vi "Get Interface Status.vi"(8 "error in (no error)":errorcluster, 11 "Application in":refnum<class "Application.lvclass">) -> (0 "error out":errorcluster, 2 "RED panel Cluster":T1={"Exposing"=TRUE, "% Acquired"=0.0, "Initialization"=FALSE, "CurrentlyTemp"=0, "Exposições realizadas"=0, "Image Graph"=[], "Temperature Status"="", "Last Image"=""} {"Exposições realizadas" scale=0.0..1.0}, 3 "Application out":refnum<class "Application.lvclass">)   [LabVIEW 2018, in "Application.lvclass"]
doc: "Este VI faz a leitura do status da interface: porcentagem de exposição da imagem atual, indicador de exposição, temperatura do CCD, indicador de inicialização do CCD, número de exposições realizadas, status da temperatura (para controle da cor do background do indicador de temperatura), última imagem obtida e gráfico da última imagem."
uses:
  Application.lvclass
  Application.lvclass/Application.ctl
  CCDCamera/CCDCamera.lvclass/CCDCamera.ctl
  Cooler/Cooler.lvclass/Cooler.ctl
  CCDCamera/CCDCamera.lvclass
  Display Image/Display Image.lvclass
  Cooler/Cooler.lvclass
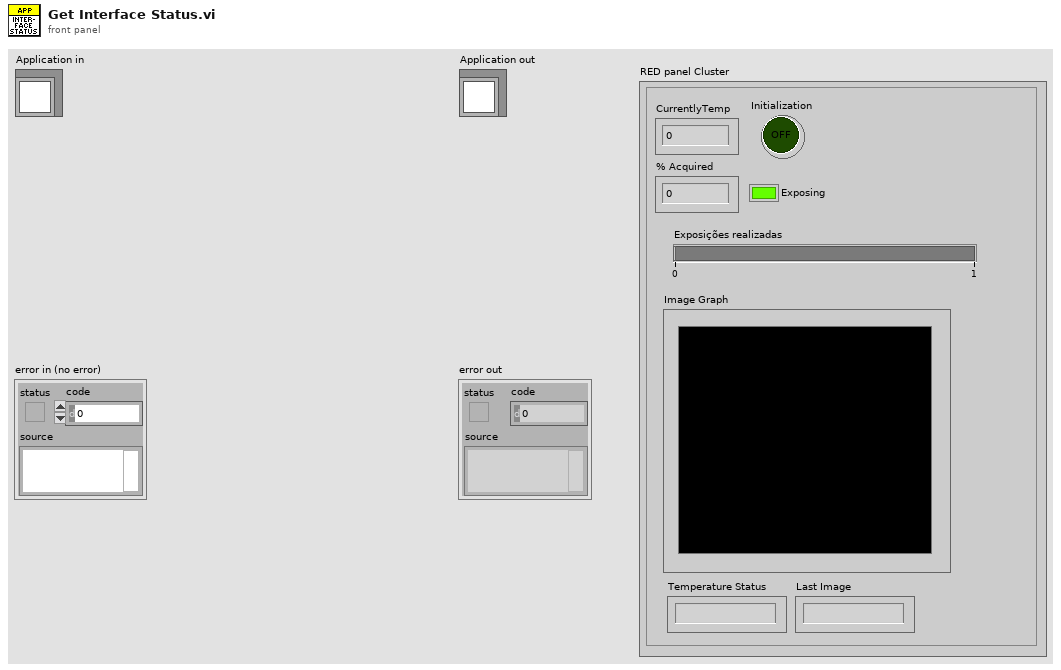
[diagram p1: front panel]
types:
  T1 = cluster{"Exposing":bool, "% Acquired":dbl, "Initialization":bool, "CurrentlyTemp":i16, "Exposições realizadas":u8, "Image Graph":i32[][], "Temperature Status":string, "Last Image":string}
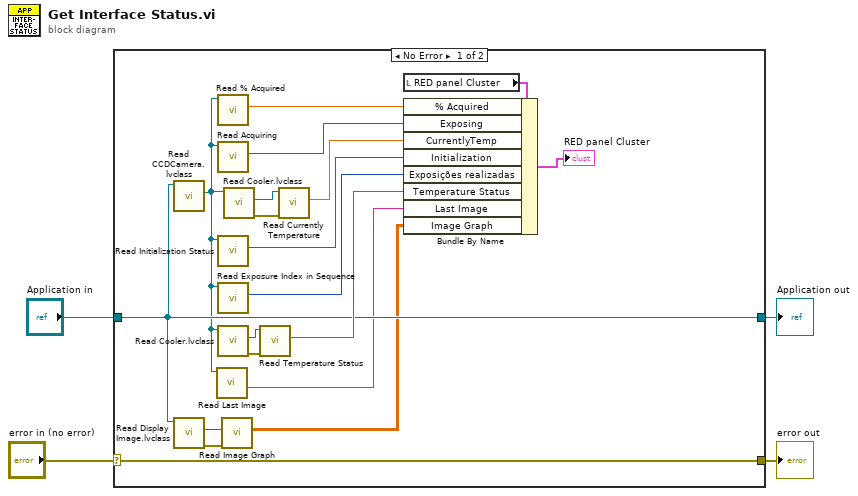
[diagram p0: block diagram]
diagram:
  n1 = case shown="No Error" "error in (no error)" {
    selector: "error in (no error)" -> [w23 w25]
    tunnel: [w23 w25] -> w3
    tunnel: [w10 w24] -> w1
    tunnel: "Application in" -> [w10 w24]
    frame No Error {
      n2 = call "Read CCDCamera.lvclass.vi"("Application in"=w10) -> ("CCDCamera.lvclass"=w6:refnum<class "CCDCamera.lvclass">)  [unwired: 8 in, 2 out]
      n3 = call "Read Display Image.lvclass.vi"("Application in"=w10) -> ("error out"=w9:errorcluster, "Display Image.lvclass"=w8:refnum<class "Display Image.lvclass">)  [unwired: 8 in, 1 out]
      n4 = call "Read Last Image.vi"("CCDCamera in"=w6) -> ("Last Image"=w5:string)  [unwired: 7 in, 3 out]
      n5 = call "Read % Acquired.vi"("CCDCamera in"=w6) -> ("% Acquired"=w21:dbl)  [unwired: 8 in, 2 out]
      n6 = call "Read Acquiring.vi"("CCDCamera in"=w6) -> ("Acquiring"=w20:bool)  [unwired: 8 in, 2 out]
      n7 = call "Read Initialization Status.vi"("CCDCamera in"=w6) -> ("Initialization Status"=w19:bool)  [unwired: 8 in, 2 out]
      n8 = call "Read Exposure Index in Sequence.vi"("CCDCamera in"=w6) -> ("Exposure Index in Sequence"=w17:u16)  [unwired: 8 in, 2 out]
      n9 = call "Read Cooler.lvclass.vi"("CCDCamera in"=w6) -> ("error out"=w16:errorcluster, "Cooler.lvclass"=w15:refnum<class "Cooler.lvclass">)  [unwired: 8 in, 1 out]
      n10 = call "Read Image Graph.vi"("error in (no error)"=w9, "Display Image in"=w8) -> ("Image Graph"=w7:dbl[][])  [unwired: 7 in, 2 out]
      n11 = call "Read Cooler.lvclass.vi"("CCDCamera in"=w6) -> ("error out"=w13:errorcluster, "Cooler.lvclass"=w12:refnum<class "Cooler.lvclass">)  [unwired: 8 in, 1 out]
      n12 = call "Read Temperature Status.vi"("error in (no error)"=w16, "Cooler in"=w15) -> ("Temperature Status"=w14:string)  [unwired: 7 in, 2 out]
      n13 = call "Read Currently Temperature.vi"("error in (no error)"=w13, "Cooler in"=w12) -> ("Currently Temperature"=w11:dbl)  [unwired: 7 in, 2 out]
      n14 = local read "RED panel Cluster"() -> (w18:T1)
      n15 = Bundle By Name(cluster=w18, "% Acquired"=w21, "Exposing"=w20, "CurrentlyTemp"=w11, "Initialization"=w19, "Exposições realizadas"=w17, "Temperature Status"=w14, "Last Image"=w5, "Image Graph"=w7) -> (→"RED panel Cluster":T1)
    }
    frame Error {
    }
  }
  "error out" <- w3
  "Application out" <- w1
